vi "WPI_CameraCompressionMode.vi"(9 "JPEG":bool, 10 "VM Index":i32, 11 "Video Modes":T1(array[cluster])=[{"Video Mode"=0, "Video Mode Name"="640 x 480 YUY 2 30.00 fps"}, {"Video Mode"=1, "Video Mode Name"="640 x 480 YUY 2 20.00 fps"}, {"Video Mode"=2, "Video Mode Name"="640 x 480 YUY 2 15.00 fps"}, {"Video Mode"=3, "Video Mode Name"="640 x 480 YUY 2 10.00 fps"}, {"Video Mode"=4, "Video Mode Name"="640 x 480 YUY 2 7.50 fps"}, {"Video Mode"=5, "Video Mode Name"="1280 x 720 YUY 2 10.00 fps"}, {"Video Mode"=6, "Video Mode Name"="1280 x 720 YUY 2 7.50 fps"}, {"Video Mode"=7, "Video Mode Name"="960 x 544 YUY 2 15.00 fps"}, {"Video Mode"=8, "Video Mode Name"="960 x 544 YUY 2 10.00 fps"}, {"Video Mode"=9, "Video Mode Name"="960 x 544 YUY 2 7.50 fps"}, {"Video Mode"=10, "Video Mode Name"="800 x 448 YUY 2 20.00 fps"}, {"Video Mode"=11, "Video Mode Name"="800 x 448 YUY 2 15.00 fps"}, {"Video Mode"=12, "Video Mode Name"="800 x 448 YUY 2 10.00 fps"}, {"Video Mode"=13, "Video Mode Name"="800 x 448 YUY 2 7.50 fps"}, {"Video Mode"=14, "Video Mode Name"="640 x 360 YUY 2 30.00 fps"}, {"Video Mode"=15, "Video Mode Name"="640 x 360 YUY 2 20.00 fps"}, {"Video Mode"=16, "Video Mode Name"="640 x 360 YUY 2 15.00 fps"}, {"Video Mode"=17, "Video Mode Name"="640 x 360 YUY 2 10.00 fps"}, {"Video Mode"=18, "Video Mode Name"="640 x 360 YUY 2 7.50 fps"}, {"Video Mode"=19, "Video Mode Name"="424 x 240 YUY 2 30.00 fps"}, {"Video Mode"=20, "Video Mode Name"="424 x 240 YUY 2 20.00 fps"}, {"Video Mode"=21, "Video Mode Name"="424 x 240 YUY 2 15.00 fps"}, {"Video Mode"=22, "Video Mode Name"="424 x 240 YUY 2 10.00 fps"}, {"Video Mode"=23, "Video Mode Name"="424 x 240 YUY 2 7.50 fps"}, {"Video Mode"=24, "Video Mode Name"="352 x 288 YUY 2 30.00 fps"}, {"Video Mode"=25, "Video Mode Name"="352 x 288 YUY 2 20.00 fps"}, {"Video Mode"=26, "Video Mode Name"="352 x 288 YUY 2 15.00 fps"}, {"Video Mode"=27, "Video Mode Name"="352 x 288 YUY 2 10.00 fps"}, {"Video Mode"=28, "Video Mode Name"="352 x 288 YUY 2 7.50 fps"}, {"Video Mode"=29, "Video Mode Name"="320 x 240 YUY 2 30.00 fps"}, {"Video Mode"=30, "Video Mode Name"="320 x 240 YUY 2 20.00 fps"}, {"Video Mode"=31, "Video Mode Name"="320 x 240 YUY 2 15.00 fps"}, {"Video Mode"=32, "Video Mode Name"="320 x 240 YUY 2 10.00 fps"}, {"Video Mode"=33, "Video Mode Name"="320 x 240 YUY 2 7.50 fps"}, {"Video Mode"=34, "Video Mode Name"="800 x 600 YUY 2 15.00 fps"}, {"Video Mode"=35, "Video Mode Name"="800 x 600 YUY 2 10.00 fps"}, {"Video Mode"=36, "Video Mode Name"="800 x 600 YUY 2 7.50 fps"}, {"Video Mode"=37, "Video Mode Name"="176 x 144 YUY 2 30.00 fps"}, {"Video Mode"=38, "Video Mode Name"="176 x 144 YUY 2 20.00 fps"}, {"Video Mode"=39, "Video Mode Name"="176 x 144 YUY 2 15.00 fps"}, {"Video Mode"=40, "Video Mode Name"="176 x 144 YUY 2 10.00 fps"}, {"Video Mode"=41, "Video Mode Name"="176 x 144 YUY 2 7.50 fps"}, {"Video Mode"=42, "Video Mode Name"="160 x 120 YUY 2 30.00 fps"}, {"Video Mode"=43, "Video Mode Name"="160 x 120 YUY 2 20.00 fps"}, {"Video Mode"=44, "Video Mode Name"="160 x 120 YUY 2 15.00 fps"}, {"Video Mode"=45, "Video Mode Name"="160 x 120 YUY 2 10.00 fps"}, {"Video Mode"=46, "Video Mode Name"="160 x 120 YUY 2 7.50 fps"}, {"Video Mode"=47, "Video Mode Name"="1280 x 800 YUY 2 10.00 fps"}, {"Video Mode"=48, "Video Mode Name"="640 x 480 JPEG 30.00 fps"}, {"Video Mode"=49, "Video Mode Name"="640 x 480 JPEG 20.00 fps"}, {"Video Mode"=50, "Video Mode Name"="640 x 480 JPEG 15.00 fps"}, {"Video Mode"=51, "Video Mode Name"="640 x 480 JPEG 10.00 fps"}, {"Video Mode"=52, "Video Mode Name"="640 x 480 JPEG 7.50 fps"}, {"Video Mode"=53, "Video Mode Name"="1280 x 720 JPEG 30.00 fps"}, {"Video Mode"=54, "Video Mode Name"="1280 x 720 JPEG 20.00 fps"}, {"Video Mode"=55, "Video Mode Name"="1280 x 720 JPEG 15.00 fps"}, {"Video Mode"=56, "Video Mode Name"="1280 x 720 JPEG 10.00 fps"}, {"Video Mode"=57, "Video Mode Name"="1280 x 720 JPEG 7.50 fps"}, {"Video Mode"=58, "Video Mode Name"="960 x 544 JPEG 30.00 fps"}, {"Video Mode"=59, "Video Mode Name"="960 x 544 JPEG 20.00 fps"}, {"Video Mode"=60, "Video Mode Name"="960 x 544 JPEG 15.00 fps"}, {"Video Mode"=61, "Video Mode Name"="960 x 544 JPEG 10.00 fps"}, {"Video Mode"=62, "Video Mode Name"="960 x 544 JPEG 7.50 fps"}, {"Video Mode"=63, "Video Mode Name"="800 x 448 JPEG 30.00 fps"}, {"Video Mode"=64, "Video Mode Name"="800 x 448 JPEG 20.00 fps"}, {"Video Mode"=65, "Video Mode Name"="800 x 448 JPEG 15.00 fps"}, {"Video Mode"=66, "Video Mode Name"="800 x 448 JPEG 10.00 fps"}, {"Video Mode"=67, "Video Mode Name"="800 x 448 JPEG 7.50 fps"}, {"Video Mode"=68, "Video Mode Name"="640 x 360 JPEG 30.00 fps"}, {"Video Mode"=69, "Video Mode Name"="640 x 360 JPEG 20.00 fps"}, {"Video Mode"=70, "Video Mode Name"="640 x 360 JPEG 15.00 fps"}, {"Video Mode"=71, "Video Mode Name"="640 x 360 JPEG 10.00 fps"}, {"Video Mode"=72, "Video Mode Name"="640 x 360 JPEG 7.50 fps"}, {"Video Mode"=73, "Video Mode Name"="800 x 600 JPEG 30.00 fps"}, {"Video Mode"=74, "Video Mode Name"="800 x 600 JPEG 20.00 fps"}, {"Video Mode"=75, "Video Mode Name"="800 x 600 JPEG 15.00 fps"}, {"Video Mode"=76, "Video Mode Name"="800 x 600 JPEG 10.00 fps"}, {"Video Mode"=77, "Video Mode Name"="800 x 600 JPEG 7.50 fps"}, {"Video Mode"=78, "Video Mode Name"="416 x 240 JPEG 30.00 fps"}, {"Video Mode"=79, "Video Mode Name"="416 x 240 JPEG 20.00 fps"}, {"Video Mode"=80, "Video Mode Name"="416 x 240 JPEG 15.00 fps"}, {"Video Mode"=81, "Video Mode Name"="416 x 240 JPEG 10.00 fps"}, {"Video Mode"=82, "Video Mode Name"="416 x 240 JPEG 7.50 fps"}, {"Video Mode"=83, "Video Mode Name"="352 x 288 JPEG 30.00 fps"}, {"Video Mode"=84, "Video Mode Name"="352 x 288 JPEG 20.00 fps"}, {"Video Mode"=85, "Video Mode Name"="352 x 288 JPEG 15.00 fps"}, {"Video Mode"=86, "Video Mode Name"="352 x 288 JPEG 10.00 fps"}, {"Video Mode"=87, "Video Mode Name"="352 x 288 JPEG 7.50 fps"}, {"Video Mode"=88, "Video Mode Name"="176 x 144 JPEG 30.00 fps"}, {"Video Mode"=89, "Video Mode Name"="176 x 144 JPEG 20.00 fps"}, {"Video Mode"=90, "Video Mode Name"="176 x 144 JPEG 15.00 fps"}, {"Video Mode"=91, "Video Mode Name"="176 x 144 JPEG 10.00 fps"}, {"Video Mode"=92, "Video Mode Name"="176 x 144 JPEG 7.50 fps"}, {"Video Mode"=93, "Video Mode Name"="320 x 240 JPEG 30.00 fps"}, {"Video Mode"=94, "Video Mode Name"="320 x 240 JPEG 20.00 fps"}, {"Video Mode"=95, "Video Mode Name"="320 x 240 JPEG 15.00 fps"}, {"Video Mode"=96, "Video Mode Name"="320 x 240 JPEG 10.00 fps"}, {"Video Mode"=97, "Video Mode Name"="320 x 240 JPEG 7.50 fps"}, {"Video Mode"=98, "Video Mode Name"="160 x 120 JPEG 30.00 fps"}, {"Video Mode"=99, "Video Mode Name"="160 x 120 JPEG 20.00 fps"}, {"Video Mode"=100, "Video Mode Name"="160 x 120 JPEG 15.00 fps"}, {"Video Mode"=101, "Video Mode Name"="160 x 120 JPEG 10.00 fps"}, {"Video Mode"=102, "Video Mode Name"="160 x 120 JPEG 7.50 fps"}]) -> (1 "Changed":bool, 2 "VM Index out":i32)   [LabVIEW 2017]
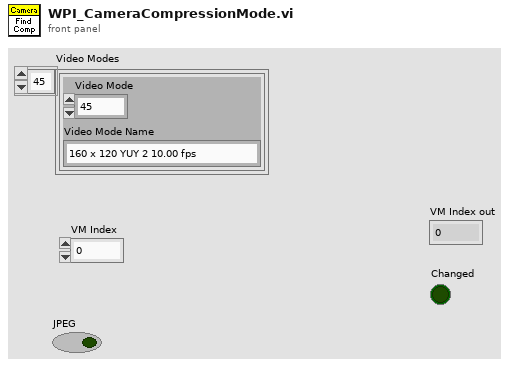
[diagram p1: front panel]
types:
  T1 = cluster{"Video Mode":u32, "Video Mode Name":string}[]
  T2 = cluster{"Video Mode":u32, "Video Mode Name":string}
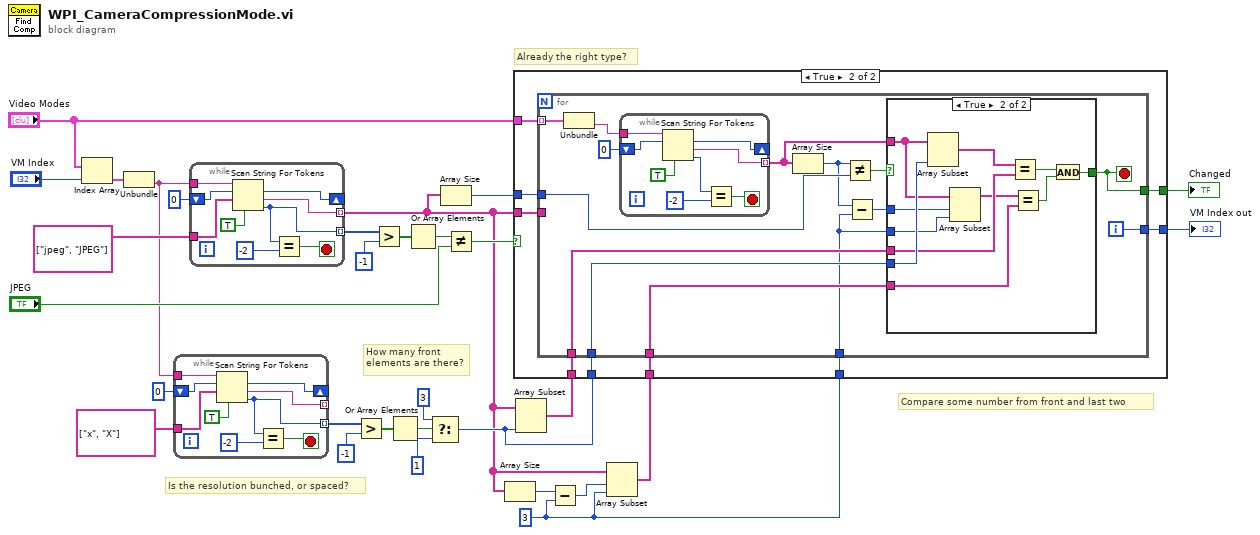
[diagram p0: block diagram]
diagram:
  w1 = 3 ("offset past token")
  # "Compare some number from front and last two"
  # "Already the right type?"
  # "Is the resolution bunched, or spaced?"
  # "How many front\nelements are there?"
  n1 = Index Array(array="Video Modes", index="VM Index") -> (element=w19:T2)
  n2 = Unbundle(w19) -> ("Video Mode Name"=w17:string)  [unwired: 1 out]
  n3 = while {
    tunnel: w17 -> [w39]
    shift-right: [w31] -> _
    shift-left: 0 ("offset past token") -> [w38]
    tunnel: [w36] -> _ mode=indexing
    tunnel: string[] ["x", "X"] -> [w33]
    tunnel: [w32] -> w13 mode=indexing
    stop <- w34 stop-if-true
    n4 = Scan String For Tokens(4:TRUE ("use cached delim/oper data? (F)"), 7:w33, 8:w38, 9:w39) -> (0:w32:i32, 1:w36:string, 2:w31:i32)  [unwired: 2 in, 1 out]
    n5 = Equal?(x=w32, y=-2) -> (x = y?=w34:bool)
  }
  n6 = while {
    tunnel: w17 -> [w48]
    shift-right: [w40] -> _
    shift-left: 0 ("offset past token") -> [w47]
    tunnel: [w45] -> w6 mode=indexing
    tunnel: string[] ["jpeg", "JPEG"] -> [w42]
    tunnel: [w41] -> w25 mode=indexing
    stop <- w43 stop-if-true
    n7 = Scan String For Tokens(4:TRUE ("use cached delim/oper data? (F)"), 7:w42, 8:w47, 9:w48) -> (0:w41:i32, 1:w45:string, 2:w40:i32)  [unwired: 2 in, 1 out]
    n8 = Equal?(x=w41, y=-2) -> (x = y?=w43:bool)
  }
  n9 = Greater?(x=w13, y=-1 ("offset past token")) -> (0:w15:bool[])
  n10 = Greater?(x=w25, y=-1 ("offset past token")) -> (0:w23:bool[])
  n11 = Or Array Elements(Boolean array=w15) -> (logical OR=w12:bool)
  n12 = Or Array Elements(Boolean array=w23) -> (logical OR=w28:bool)
  n13 = Select(t=3 ("offset past token"), s=w12, f=1 ("offset past token")) -> (s? t:f=w9:i32)
  n14 = Array Size(array=w6) -> (size(s)=w22:i32)
  n15 = Not Equal?(x=w28, y="JPEG") -> (x != y?=w26:bool)
  n16 = Array Size(array=w6) -> (size(s)=w5:i32)
  n17 = Array Subset(array=w6, length=w9) -> (w8:string[])  [unwired: 1 in]
  n18 = Subtract(x=w5, y=w1) -> (x-y=w4:i32)
  n19 = Array Subset(array=w6, index=w4, length=w1) -> (w7:string[])
  n20 = case shown="True" w26 {
    tunnel: "Video Modes" -> [_ w57]
    tunnel: w6 -> [_ w55]
    tunnel: w22 -> [_ w56]
    tunnel: w9 -> [_ w54]
    tunnel: w8 -> [_ w53]
    tunnel: w7 -> [_ w52]
    tunnel: [_ w51] -> w3
    tunnel: [_ w50] -> w2
    tunnel: w1 -> [_ w49]
    frame False {
    }
    frame True {
      n21 = for {
        tunnel: w57 -> [w71] mode=indexing
        tunnel: w56 -> [w68]
        tunnel: w55 -> [_]
        tunnel: w54 -> [w65]
        tunnel: w53 -> [w64]
        tunnel: w52 -> [w61]
        tunnel: [w60] -> w51
        tunnel: [w59] -> w50
        tunnel: w49 -> [w58]
        i -> [w60]
        stop <- w59 stop-if-true
        n22 = Unbundle(w71) -> ("Video Mode Name"=w69:string)  [unwired: 1 out]
        n23 = while {
          tunnel: w69 -> [w90]
          shift-right: [w83] -> _
          shift-left: 0 ("offset past token") -> [w89]
          tunnel: [w87] -> w66 mode=indexing
          stop <- w85 stop-if-true
          n24 = Scan String For Tokens(4:TRUE ("use cached delim/oper data? (F)"), 8:w89, 9:w90) -> (0:w84:i32, 1:w87:string, 2:w83:i32)  [unwired: 3 in, 1 out]
          n25 = Equal?(x=w84, y=-2) -> (x = y?=w85:bool)
        }
        n26 = Array Size(array=w66) -> (size(s)=w63:i32)
        n27 = Not Equal?(x=w63, y=w68) -> (x != y?=w67:bool)
        n28 = Subtract(x=w63, y=w58) -> (x-y=w62:i32)
        n29 = case shown="True" w67 {
          tunnel: w66 -> [_ w77]
          tunnel: w65 -> [_ w82]
          tunnel: w64 -> [_ w80]
          tunnel: w58 -> [_ w76]
          tunnel: w62 -> [_ w75]
          tunnel: w61 -> [_ w73]
          tunnel: [_ w72] -> w59
          frame False {
          }
          frame True {
            n30 = Array Subset(array=w77, length=w82) -> (w81:string[])  [unwired: 1 in]
            n31 = Array Subset(array=w77, index=w75, length=w76) -> (w74:string[])
            n32 = Equal?(x=w81, y=w80) -> (x = y?=w78:bool)
            n33 = Equal?(x=w74, y=w73) -> (x = y?=w79:bool)
            n34 = And(x=w78, y=w79) -> (x .and. y?=w72:bool)
          }
        }
      }
    }
  }
  "VM Index out" <- w3
  "Changed" <- w2
